vi "NCS_IQ.vi"(0 "Tone Amplitude":dbl, 1 "Waveform Size":dbl, 2 "Tone Frequency":dbl, 3 "Coerced IQ rate":dbl, 5 "error in (no error)":errorcluster) -> (6 "IQ waveform":waveform(dbl)[](array[waveform]), 7 "IQ waveform array":cdb[](array[numeric]), 8 "error out":errorcluster)   [LabVIEW 2016]
uses:
  <vilib>/measure/NI_MABase.lvlib
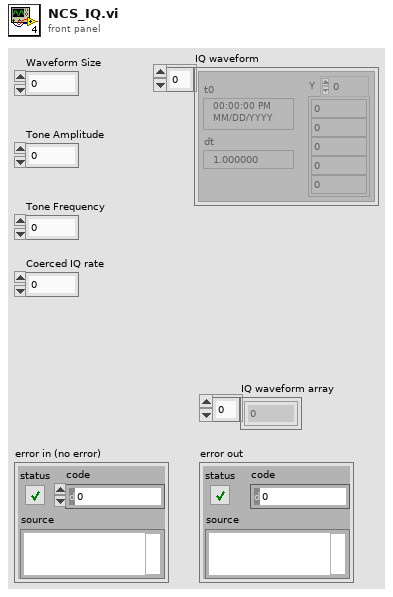
[diagram p1: front panel]
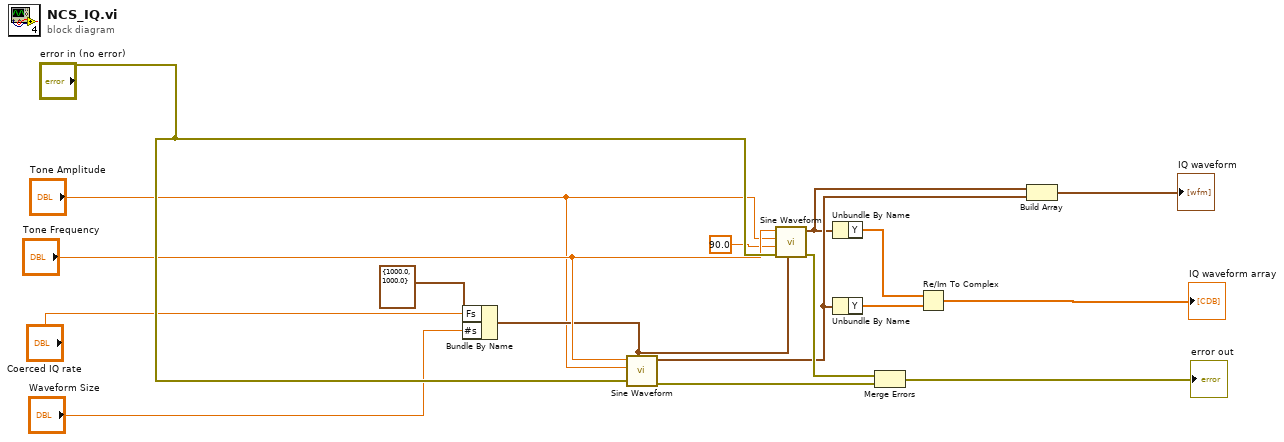
[diagram p0: block diagram]
diagram:
  n1 = Bundle By Name(cluster=cluster{"Fs":dbl, "#s":dbl} {"Fs"=1000.0, "#s"=1000.0} ("sampling info"), "Fs"="Coerced IQ rate", "#s"="Waveform Size") -> (w11:cluster{"Fs":dbl, "#s":dbl})
  n2 = call <vilib>:"Sine Waveform.vi"("sampling info"=w11, "error in (no error)"="error in (no error)", "amplitude"="Tone Amplitude", "frequency"="Tone Frequency") -> ("error out"=w12:errorcluster, "signal out"=w3:waveform(dbl))  [unwired: 6 in]
  n3 = call <vilib>:"Sine Waveform.vi"("sampling info"=w11, "error in (no error)"="error in (no error)", "phase"=90.0, "amplitude"="Tone Amplitude", "frequency"="Tone Frequency") -> ("error out"=w13:errorcluster, "signal out"=w2:waveform(dbl))  [unwired: 5 in]
  n4 = Unbundle By Name(w2) -> ("Y"=w6:dbl[])
  n5 = Unbundle By Name(w3) -> ("Y"=w7:dbl[])
  n6 = Merge Errors(w13, w12) -> (→"error out":errorcluster)
  n7 = Re/Im To Complex(1:w7, 2:w6) -> (0:→"IQ waveform array":cdb[])
  n8 = Build Array(w2, w3) -> (→"IQ waveform":waveform(dbl)[])
